vi "setAxisGrid.vi"(7 "Grids":T3, 8 "polarGridAngle":dbl, 9 "Axis":T2="x", 11 "String in":string) -> (3 "String out":string)   [LabVIEW 2013]
uses:
  grids.ctl
  axisName.ctl
  commandArray.ctl
panel:
  out "Commands":T1
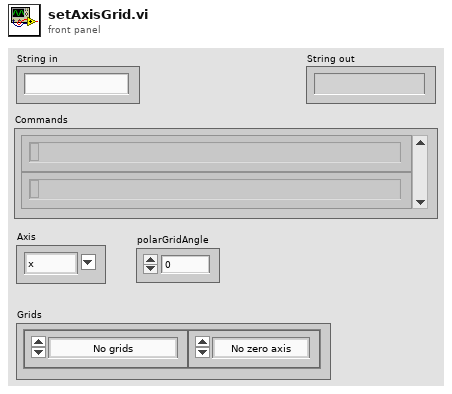
[diagram p1: front panel]
types:
  T1 = typedef "commandArray.ctl" = string[]
  T2 = typedef "axisName.ctl" = string
  T3 = typedef "grids.ctl" = cluster{"Gridlines":enum16{"No grids", "Major grid", "Minor grid", "Major and Minor"}, "Zeroaxis":enum16{"No zero axis", "Show zero axis"}}
  T4 = enum16{"No grids", "Major grid", "Minor grid", "Major and Minor"}
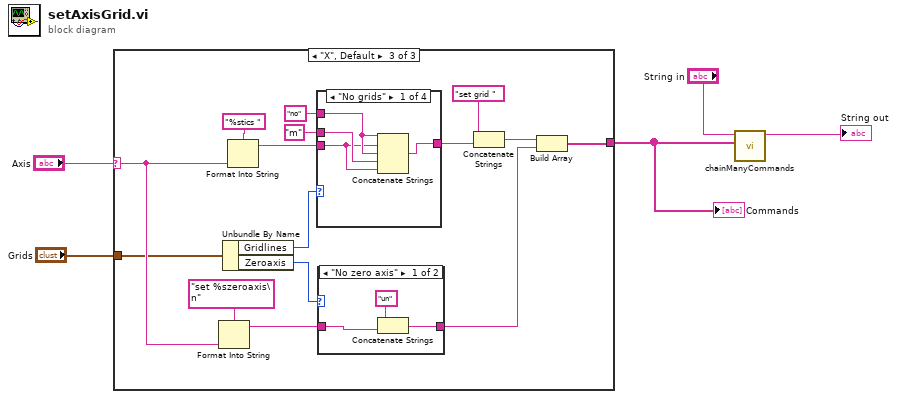
[diagram p0: block diagram]
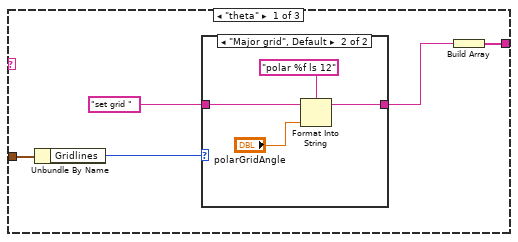
[diagram p2: hidden frame]
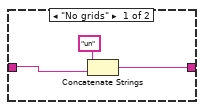
[diagram p3: hidden frame]
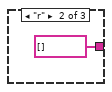
[diagram p4: hidden frame]
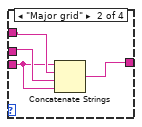
[diagram p6: hidden frame]
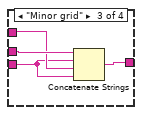
[diagram p7: hidden frame]
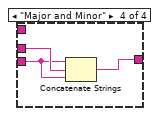
[diagram p8: hidden frame]
diagram:
  n1 = case shown="\"X\", Default" "Axis" {
    selector: "Axis" -> [_ _ w23]
    tunnel: [w7 string[] [] w20] -> w2
    tunnel: "Grids" -> [w10 _ w22]
    frame "theta" {
      n2 = Unbundle By Name(w10) -> ("Gridlines"=w8:T4)
      n3 = case shown="\"Major grid\", Default" w8 {
        tunnel: [w13 w15] -> w6
        tunnel: "set grid " ("initial string") -> [w12 w14]
        frame "No grids" {
          n4 = Concatenate Strings("un" ("string"), w12) -> (w13:string)
        }
        frame "Major grid", Default {
          n5 = Format Into String(format string="polar %f ls 12", initial string=w14, "polarGridAngle") -> (resulting string=w15:string)  [unwired: 1 in, 1 out]
        }
      }
      n6 = Build Array(w6) -> (w7:string[])
    }
    frame "r" {
    }
    frame "X", Default {
      n7 = Format Into String(format string="set %szeroaxis\n", w23) -> (resulting string=w24:string)  [unwired: 2 in, 1 out]
      n8 = Unbundle By Name(w22) -> ("Gridlines"=w32:T4, "Zeroaxis"=w31:enum16{"No zero axis", "Show zero axis"})
      n9 = Format Into String(format string="%stics ", w23) -> (resulting string=w28:string)  [unwired: 2 in, 1 out]
      n10 = case shown="\"No grids\"" w32 {
        tunnel: [w41 w45 w49 w50] -> w33
        tunnel: w28 -> [w38 w42 w46 w51]
        tunnel: "no" ("format string") -> [w40 w44 w47 _]
        tunnel: "m" ("format string") -> [w39 w43 w48 w52]
        frame "No grids" {
          n11 = Concatenate Strings(w40, w38, w40, w39, w38) -> (w41:string)
        }
        frame "Major grid" {
          n12 = Concatenate Strings(w42, w44, w43, w42) -> (w45:string)
        }
        frame "Minor grid" {
          n13 = Concatenate Strings(w48, w46, w47, w46) -> (w49:string)
        }
        frame "Major and Minor" {
          n14 = Concatenate Strings(w51, w52, w51) -> (w50:string)
        }
      }
      n15 = case shown="\"No zero axis\"" w31 {
        tunnel: [w36 w37] -> w19
        tunnel: w24 -> [w35 w37]
        frame "No zero axis" {
          n16 = Concatenate Strings("un", w35) -> (w36:string)
        }
        frame "Show zero axis" {
        }
      }
      n17 = Concatenate Strings("set grid ", w33) -> (w21:string)
      n18 = Build Array(w21, w19) -> (w20:string[])
    }
  }
  "Commands" <- w2
  n19 = call "chainManyCommands.vi"("CommandArray"=w2, "String in in"="String in") -> ("String out"=→"String out":string)  [unwired: 9 in]
